vi "GT Set Trigger.vi"(8 "error in (no error)":errorcluster caption="错误输入（无错误）", 9 "pTrigger":T1, 10 "i":i16, 11 "cardNum":i16) -> (0 "error out":errorcluster caption="错误输出", 1 "pTrigger out":T1, 3 "function return":i16)   [LabVIEW 2020, in "gts.lvlib"]
doc: "GT_API GT_SetTrigger(short cardNum,short i,TTrigger *pTrigger);"
uses:
  gts.lvlib
  dll/32bit/multi_card/gts.dll
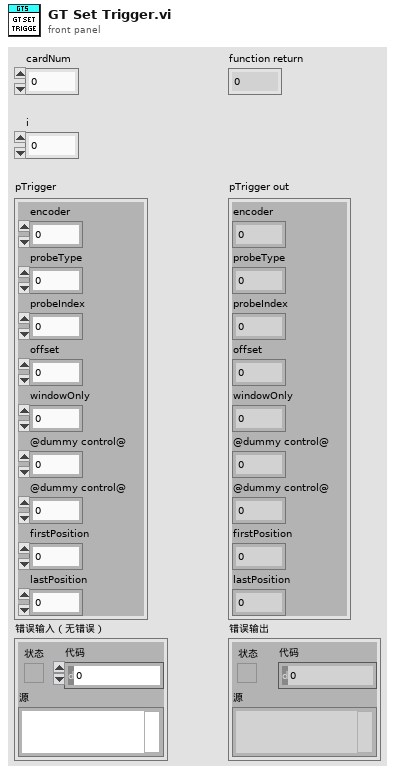
[diagram p1: front panel]
types:
  T1 = cluster{"encoder":i16, "probeType":i16, "probeIndex":i16, "offset":i16, "windowOnly":i16, "@dummy control@":i8, "@dummy control@":i8, "firstPosition":i32, "lastPosition":i32}
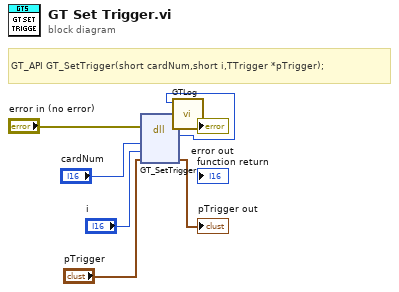
[diagram p0: block diagram]
diagram:
  # "GT_API GT_SetTrigger(short cardNum,short i,TTrigger *pTrigger);"
  n1 = dll-call lib="C:/1228/dll/32bit/multi_card/gts.dll" fn="GT_SetTrigger"(error in="error in (no error)", "cardNum"="cardNum", "i"="i", "pTrigger"="pTrigger") -> (error out=w3:errorcluster, w1:i16, "pTrigger"=→"pTrigger out":T1)  [unwired: 4 in, 1 out]
  n2 = call "GTLog.vi"("error in (no error)"=w3, "Numeric"=w1) -> ("error out"=→"error out":errorcluster)  [unwired: 9 in]
